vi "DeviceInfo2Str.vi"(11 "Device Information":string[](array[string])) -> (3 "String":string)   [LabVIEW 2020]
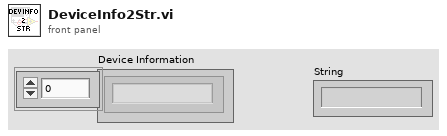
[diagram p1: front panel]
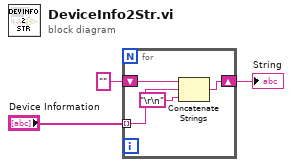
[diagram p0: block diagram]
diagram:
  n1 = for {
    tunnel: "Device Information" -> [w6] mode=indexing
    shift-right: [w4] -> w1
    shift-left: "" -> [w7]
    n2 = Concatenate Strings(w7, w6, "\r\n") -> (w4:string)
  }
  "String" <- w1
